vi "TimeInterpRotation2d_GetNewestSample.vi"(11 "TimeInterpRotation2d":T1 {"RotationValues"."SIN" format="%13.4f"; "RotationValues"."COS" format="%13.4f"; "RotationValues"."VALUE" format="%13.4f"}) -> (1 "IsPresent":bool, 2 "TimeStamp":dbl, 3 "OutputRotation2d":T2={"VALUE"=0.0, "COS"=1.0, "SIN"=0.0} {"SIN" format="%13.4f"; "COS" format="%13.4f"; "VALUE" format="%13.4f"})   [LabVIEW 2019, in "Trajectory_Library.lvlib"]
doc: "Get the newest sample\n\nInputs:\n - TimeInterpRotatin2d -- Input data cluster\n\nOutputs\n - OutputRotatin2d -- Newest Rotation2d. \n - TimeStamp -- Time for this sample (seconds)\n - IsPresent -- Returns TRUE if the buffer contains any data"
uses:
  Trajectory_Library.lvlib
  TypeDef/ROTATION2D.ctl
  TypeDef/TIME_INTERPOLATABLE_ROTATION2D.ctl
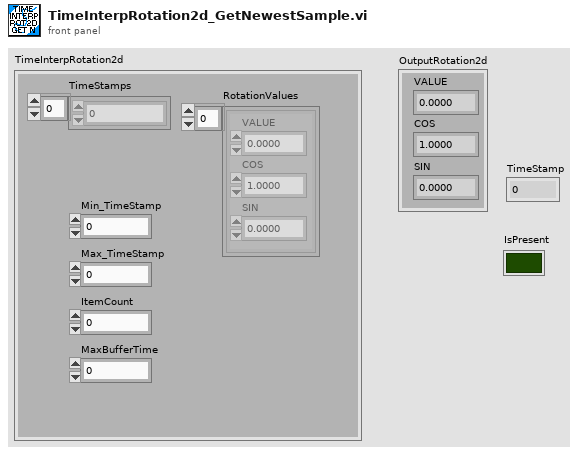
[diagram p1: front panel]
types:
  T1 = typedef "Trajectory_Library.lvlib/TIME_INTERPOLATABLE_ROTATION2D.ctl" = cluster{"TimeStamps":dbl[], "RotationValues":T2[], "Min_TimeStamp":dbl, "Max_TimeStamp":dbl, "ItemCount":i32, "MaxBufferTime":dbl}
  T2 = typedef "Trajectory_Library.lvlib/ROTATION2D.ctl" = cluster{"VALUE":dbl, "COS":dbl, "SIN":dbl}
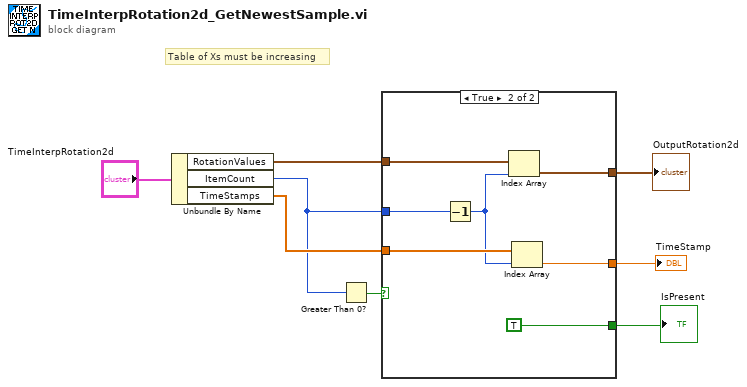
[diagram p0: block diagram]
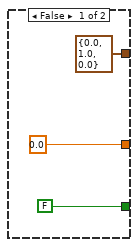
[diagram p2: hidden frame]
diagram:
  # "Table of Xs must be increasing"
  n1 = Unbundle By Name("TimeInterpRotation2d") -> ("RotationValues"=w6:T2[], "ItemCount"=w4:i32, "TimeStamps"=w7:dbl[])
  n2 = Greater Than 0?(x=w4) -> (x > 0?=w5:bool)
  n3 = case shown="True" w5 {
    tunnel: [T2 {"VALUE"=0.0, "COS"=1.0, "SIN"=0.0} ("Table Y") w15] -> w2
    tunnel: w4 -> [_ w13]
    tunnel: w7 -> [_ w17]
    tunnel: w6 -> [_ w18]
    tunnel: [FALSE TRUE] -> w3
    tunnel: [0.0 w16] -> w1
    frame False {
    }
    frame True {
      n4 = Decrement(x=w13) -> (x-1=w12:i32)
      n5 = Index Array(array=w18, index=w12) -> (element=w15:T2)
      n6 = Index Array(array=w17, index=w12) -> (element=w16:dbl)
    }
  }
  "OutputRotation2d" <- w2
  "IsPresent" <- w3
  "TimeStamp" <- w1
